vi "KepcoDCPwr Initialize With Options.vi"(0 "VISA resource name":refnum<visa-resource-name>, 1 "option string (\"Simulate=0,RangeCheck=1,QueryInstrStatus=1,Cache=1\")":string="Simulate=0,RangeCheck=1,QueryInstrStatus=1,Cache=1", 2 "recognize device (True)":bool=TRUE caption="Recognize Device (True)", 5 "Model":string, 7 "id query (True)":bool=TRUE, 9 "reset device (True)":bool=TRUE, 11 "error in (no error)":errorcluster {"code" format="%.0x"}) -> (4 "VISA Session Out":refnum<visa-resource-name>, 6 "Model Out":string, 12 "Raw Model":string, 14 "Raw idn string":string, 15 "error out":errorcluster {"code" format="%.0x"})   [LabVIEW 2013]
doc: "This VI performs the following initialization actions:\n\n- Creates a new IVI instrument driver and optionally sets the initial state of the following session properties:\n\n kpbop>>Inherent IVI Settings>>User Options>>Range Check \n KPBOP_ATTR_QUERY_INSTR_STATUS \n kpbop>>Inherent IVI Settings>>User Options>>Cache \n kpbop>>Inherent IVI Settings>>User Options>>Simulate \n kpbop>>Inherent IVI Settings>>User Options>>Record Value Coercions \n\n- Opens a session to the specified device using the interface and address you specify for the Resource Name parameter.\n\n- If the ID Query parameter is set to TRUE, this VI queries the instrument ID and checks that it is valid for this instrument driver.\n\n- If the Reset parameter is set to TRUE, this VI resets the instrument to a known state.\n\n- Sends initialization commands to set the instrument to the state necessary for the operation of the instrument driver.\n\n- Returns an instrument handle that you use to identify the instrument in all subsequent instrument driver VI calls.\n\n\n- This function must be used inorder to properly establish the model string. It has pop-ups to provide informaiton if the driver will not operate with the specific instrument at the channel address. \nNote: This VI creates a new session each time you invoke it. Although you can open more than one VISA session for the same resource, it is best not to do so. You can use the same session in multiple program threads."
uses:
  <vilib>/regexp/Match Regular Expression.xnode
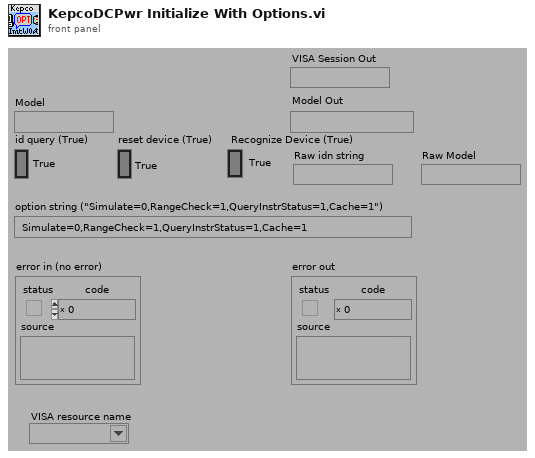
[diagram p1: front panel]
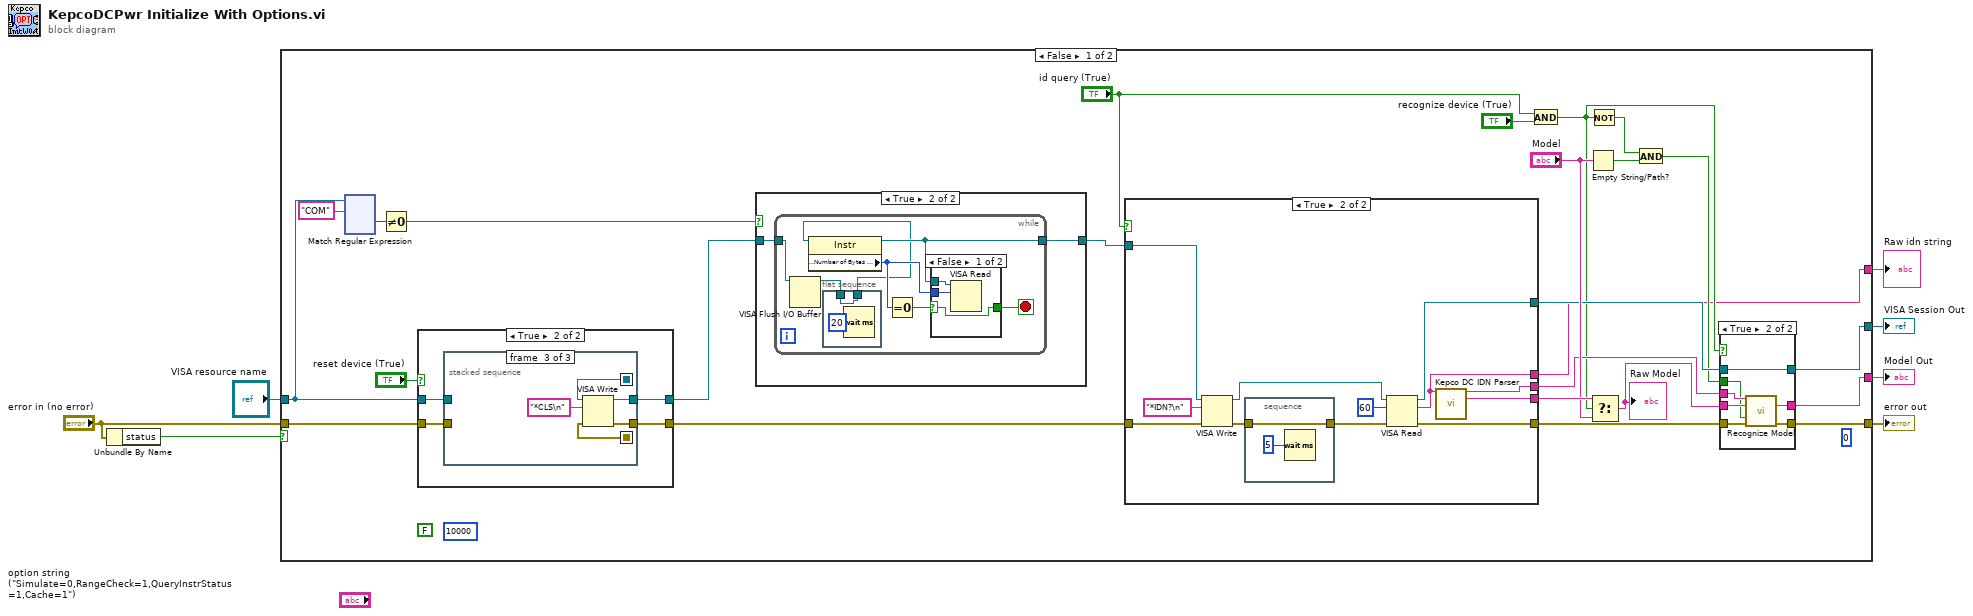
[diagram p0: block diagram]
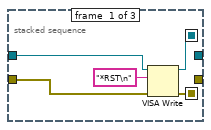
[diagram p5: hidden frame]
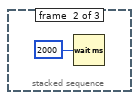
[diagram p6: hidden frame]
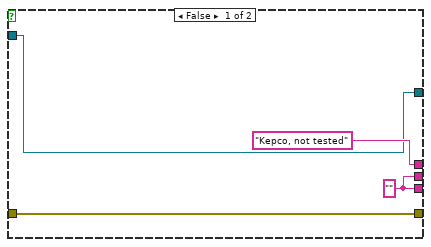
[diagram p8: hidden frame]
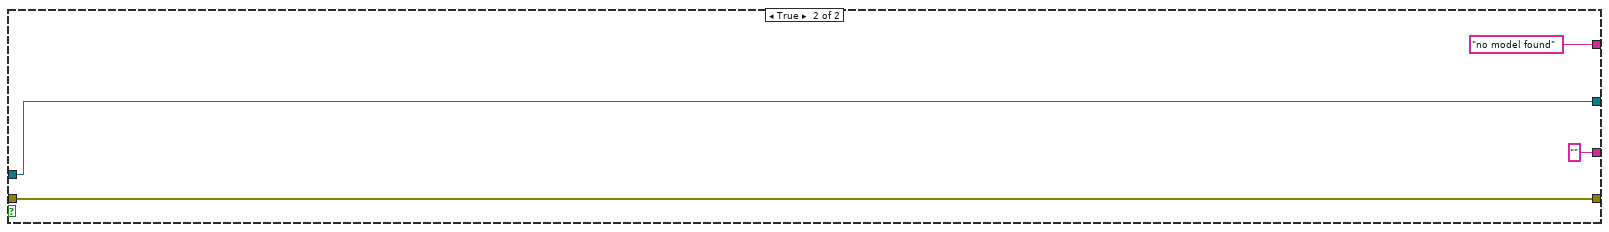
[diagram p9: hidden frame]
diagram:
  n1 = Unbundle By Name("error in (no error)") -> ("status"=w6:bool)
  n2 = case shown="False" w6 {
    tunnel: [w25 w208] -> w4
    tunnel: "error in (no error)" -> [w17 w208]
    tunnel: [w26 w206] -> w3
    tunnel: [w28 "" ("Model")] -> w5
    tunnel: "VISA resource name" -> [w13 w206]
    tunnel: [w16 "no model found" ("read buffer")] -> w1
    frame False {
      (unwired) FALSE
      (unwired) u32 10000 ("timeout (0)")
      (unwired) u32 0 ("access mode")
      n3 = xnode "Match Regular Expression"("input string"=w13, "regular expression"="COM") -> ("offset past match"=w12:i32)  [unwired: 2 in, 6 out]
      n4 = Not Equal To 0?(x=w12) -> (x != 0?=w11:bool)
      n5 = case shown="True" "reset device (True)" {
        tunnel: w13 -> [w161 w165]
        tunnel: [w161 w162] -> w8
        tunnel: w17 -> [w160 w164]
        tunnel: [w160 w163] -> w18
        frame False {
        }
        frame True {
          n6 = stacked-sequence {
            seq-local: [w167 _ _] -> [_ _ w172]
            seq-local: [w166 _ _] -> [_ _ w173]
            tunnel: w165 -> [w169 _ _]
            tunnel: [_ _ w176] -> w162
            tunnel: w164 -> [w168 _ _]
            tunnel: [_ _ w174] -> w163
            frame #0 {
              n7 = VISA Write(VISA resource name=w169, write buffer="*RST\n" ("write buffer (\"\")"), error in (no error)=w168) -> (VISA resource name out=w166:refnum<visa-resource-name>, error out=w167:errorcluster)  [unwired: 1 out]
            }
            frame #1 {
              n8 = Wait (ms)(milliseconds to wait=u32 2000) -> ()  [unwired: 1 out]
            }
            frame #2 {
              n9 = VISA Write(VISA resource name=w173, write buffer="*CLS\n" ("write buffer (\"\")"), error in (no error)=w172) -> (VISA resource name out=w176:refnum<visa-resource-name>, error out=w174:errorcluster)  [unwired: 1 out]
            }
          }
        }
      }
      n10 = case shown="True" w11 {
        tunnel: w8 -> [w33 w35]
        tunnel: [w33 w34] -> w9
        frame False {
        }
        frame True {
          n11 = while {
            tunnel: w35 -> [w38]
            tunnel: [w40] -> w34
            stop <- w41 stop-if-true
            n12 = VISA Flush I/O Buffer(VISA resource name=w38) -> (VISA resource name out=w37:refnum<visa-resource-name>)  [unwired: 2 in, 1 out]
            n13 = property class="Instr"(reference=w36) -> (reference out=w40:refnum<visa-resource-name>, "Serial Settings:Number of Bytes at Serial Port"=w39:u32)  [unwired: 1 in, 1 out]
            n14 = flat-sequence {
              tunnel: w37 -> [w43]
              tunnel: [w43] -> w36
              frame #0 {
                n15 = Wait (ms)(milliseconds to wait=u32 20) -> ()  [unwired: 1 out]
              }
            }
            n16 = Equal To 0?(x=w39) -> (x = 0?=w42:bool)
            n17 = case shown="False" w42 {
              selector: w42 -> [w47 w48]
              tunnel: [w47 w48] -> w41
              tunnel: w40 -> [w46 _]
              tunnel: w39 -> [w45 _]
              frame False {
                n18 = VISA Read(VISA resource name=w46, byte count=w45) -> ()  [unwired: 1 in, 4 out]
              }
              frame True {
              }
            }
          }
        }
      }
      n19 = case shown="True" "id query (True)" {
        tunnel: [w187 w201] -> w29
        tunnel: w18 -> [w190 w200]
        tunnel: [w190 w199] -> w30
        tunnel: [w189 w197] -> w32
        tunnel: [w189 w196] -> w27
        tunnel: ["Kepco, not tested" ("read buffer") w192] -> w16
        tunnel: w9 -> [w187 w191]
        frame False {
          w189 = "" ("Model")
        }
        frame True {
          n20 = VISA Write(VISA resource name=w191, write buffer="*IDN?\n" ("write buffer (\"\")"), error in (no error)=w200) -> (VISA resource name out=w202:refnum<visa-resource-name>, error out=w195:errorcluster)  [unwired: 1 out]
          n21 = stacked-sequence {
            tunnel: w195 -> [w204]
            tunnel: [w204] -> w194
            frame #0 {
              n22 = Wait (ms)(milliseconds to wait=u32 5) -> ()  [unwired: 1 out]
            }
          }
          n23 = VISA Read(VISA resource name=w202, byte count=u32 60 ("byte count (0)"), error in (no error)=w194) -> (VISA resource name out=w201:refnum<visa-resource-name>, read buffer=w192:string, error out=w199:errorcluster)  [unwired: 1 out]
          n24 = call "Kepco DC IDN Parser.vi"("IDN Query"=w192) -> ("Manufacturer"=w196:string, "Model"=w197:string)  [unwired: 13 out]
        }
      }
      n25 = And(x="id query (True)", y="recognize device (True)") -> (x .and. y?=w19:bool)
      n26 = Empty String/Path?(string/path="Model") -> (empty?=w22:bool)
      n27 = Not(x=w19) -> (.not. x?=w20:bool)
      n28 = Select(t=w32, s=w19, f="Model") -> (s? t:f=w15:string)
      "Raw Model" <- w15
      n29 = And(x=w20, y=w22) -> (x .and. y?=w21:bool)
      n30 = case shown="True" w19 {
        tunnel: w15 -> [w179 w185]
        tunnel: w30 -> [w178 w182]
        tunnel: w29 -> [w177 w186]
        tunnel: [w179 w184] -> w28
        tunnel: [w178 w181] -> w25
        tunnel: [w177 w186] -> w26
        tunnel: w27 -> [_ w183]
        tunnel: w21 -> [_ w180]
        frame False {
        }
        frame True {
          n31 = call "Recognize Model.vi"("Manufacturer"=w183, "Model"=w185, "Model Unwired/Wired"=w180, "error in (no error)"=w182) -> ("Model Out"=w184:string, "error out"=w181:errorcluster)  [unwired: 10 out]
        }
      }
    }
    frame True {
    }
  }
  "error out" <- w4
  "VISA Session Out" <- w3
  "Model Out" <- w5
  "Raw idn string" <- w1
